vi "Easy XML Editor Menu.vi"(8 "error in (no error)":errorcluster, 11 "Menu Refnum In":refnum<k9>) -> (0 "error out":errorcluster, 3 "Menu Refnum Out":refnum<k9>)   [LabVIEW 2017]
uses:
  <vilib>/Utility/miscctls.llb/LVMenuShortCut.ctl
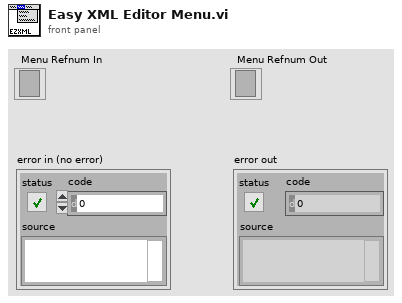
[diagram p1: front panel]
types:
  T1 = typedef "LVMenuShortCut.ctl" = cluster{"Include Shift Key?":bool, "Include Ctrl Key?":bool, "Shortcut Key":string}
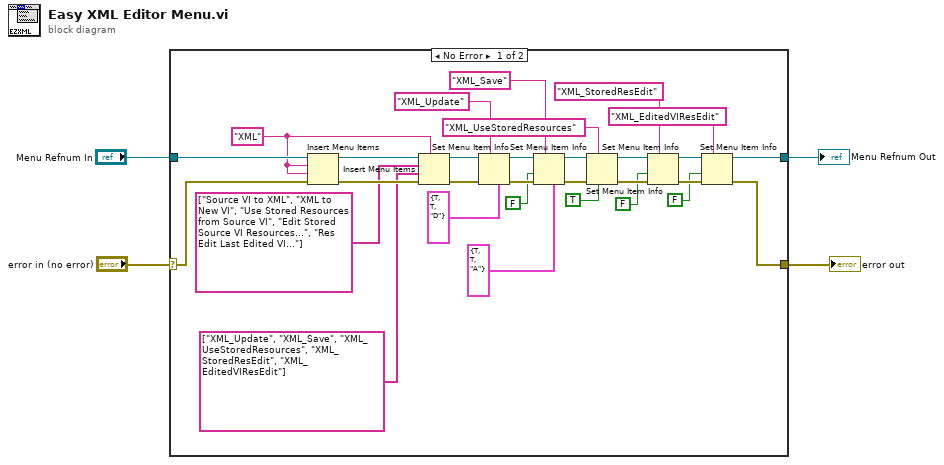
[diagram p0: block diagram]
diagram:
  n1 = case shown="No Error" "error in (no error)" {
    selector: "error in (no error)" -> [w13 w36]
    tunnel: "Menu Refnum In" -> [w34 w35]
    tunnel: [w8 w35] -> w1
    tunnel: [w7 w36] -> w2
    frame No Error {
      w21 = "XML"
      n2 = Insert Menu Items(6:w13, 7:w21, 8:w21, 9:w34) -> (0:w32:errorcluster, 3:w33:refnum<k9>)  [unwired: 2 in, 1 out]
      n3 = Insert Menu Items(5:w21, 6:w32, 7:string[] ["XML_Update", "XML_Save", "XML_UseStoredResources", "XML_StoredResEdit", "XML_EditedVIResEdit"] ("item tags"), 8:string[] ["Source VI to XML", "XML to New VI", "Use Stored Resources from Source VI", "Edit Stored Source VI Resources...", "Res Edit Last Edited VI..."] ("item names"), 9:w33) -> (0:w28:errorcluster, 3:w29:refnum<k9>)  [unwired: 1 in, 1 out]
      n4 = Set Menu Item Info(4:T1 {"Include Shift Key?"=TRUE, "Include Ctrl Key?"=TRUE, "Shortcut Key"="D"} ("short cut"), 7:"XML_Update", 8:w28, 11:w29) -> (0:w26:errorcluster, 3:w25:refnum<k9>)  [unwired: 3 in]
      n5 = Set Menu Item Info(4:T1 {"Include Shift Key?"=TRUE, "Include Ctrl Key?"=TRUE, "Shortcut Key"="A"} ("short cut"), 7:"XML_Save", 8:w26, 9:FALSE, 11:w25) -> (0:w20:errorcluster, 3:w19:refnum<k9>)  [unwired: 2 in]
      n6 = Set Menu Item Info(6:TRUE, 7:"XML_UseStoredResources" ("item tag"), 8:w20, 11:w19) -> (0:w16:errorcluster, 3:w15:refnum<k9>)  [unwired: 3 in]
      n7 = Set Menu Item Info(7:"XML_StoredResEdit", 8:w16, 9:FALSE, 11:w15) -> (0:w12:errorcluster, 3:w11:refnum<k9>)  [unwired: 3 in]
      n8 = Set Menu Item Info(7:"XML_EditedVIResEdit", 8:w12, 9:FALSE, 11:w11) -> (0:w7:errorcluster, 3:w8:refnum<k9>)  [unwired: 3 in]
    }
    frame Error {
    }
  }
  "Menu Refnum Out" <- w1
  "error out" <- w2
